vi "Configure Statistics.vi"(0 "VISA resource name":refnum<visa-resource-name>, 7 "Math Format (0: None)":u16(ring) items=["None", "Mean", "Standard Deviation", "Maximum", "Minimum", "Peak to Peak"], 11 "error in (no error)":errorcluster) -> (4 "VISA resource name out":refnum<visa-resource-name>, 15 "error out":errorcluster)   [LabVIEW 2020, in "Keithley 27XX.lvlib"]
doc: "This VI configures calculations done on the data buffer to achieve various statistical analyses."
uses:
  Keithley 27XX.lvlib
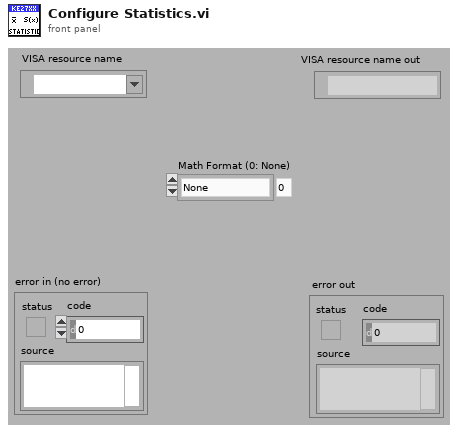
[diagram p1: front panel]
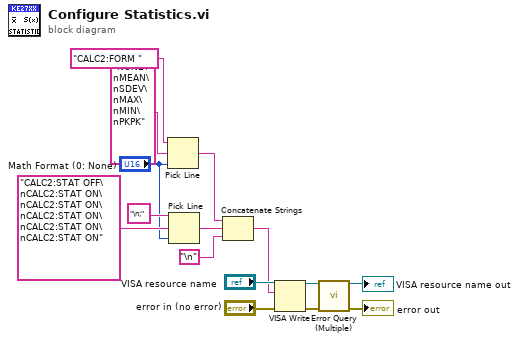
[diagram p0: block diagram]
diagram:
  n1 = Pick Line(string ("")="CALC2:FORM ", multi-line string="NONE\nMEAN\nSDEV\nMAX\nMIN\nPKPK", line index="Math Format (0: None)") -> (output string=w13:string)
  n2 = Pick Line(string ("")="\n;", multi-line string="CALC2:STAT OFF\nCALC2:STAT ON\nCALC2:STAT ON\nCALC2:STAT ON\nCALC2:STAT ON\nCALC2:STAT ON", line index="Math Format (0: None)") -> (output string=w4:string)
  n3 = Concatenate Strings(w13, w4, "\n") -> (w10:string)
  n4 = VISA Write(VISA resource name="VISA resource name", write buffer=w10, error in (no error)="error in (no error)") -> (VISA resource name out=w9:refnum<visa-resource-name>, error out=w8:errorcluster)  [unwired: 1 out]
  n5 = call "Error Query (Multiple).vi"("VISA resource name"=w9, "error in (no error)"=w8) -> ("VISA resource name out"=→"VISA resource name out":refnum<visa-resource-name>, "error out"=→"error out":errorcluster)  [unwired: 10 in, 2 out]
